vi "get_total_number_of_lines_per_frame.vi"(8 "error in (no error)":errorcluster, 11 "TrajectoryAK101022Resonance in":refnum<class "TrajectoryAK101022Resonance.lvclass">) -> (0 "error out":errorcluster, 2 "total number of lines per frame":i32, 3 "TrajectoryAK101022Resonance out":refnum<class "TrajectoryAK101022Resonance.lvclass">)   [LabVIEW 2010, in "TrajectoryAK101022Resonance.lvclass"]
uses:
  TrajectoryAK101022Resonance.lvclass
  TrajectoryAK101022Resonance.lvclass/TrajectoryAK101022Resonance.ctl
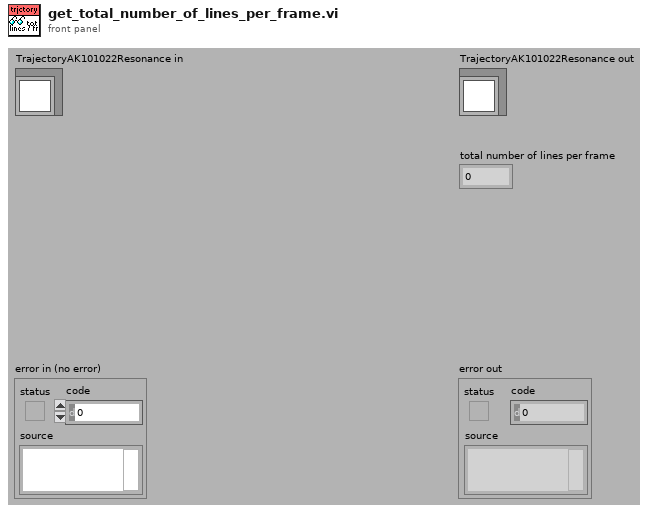
[diagram p1: front panel]
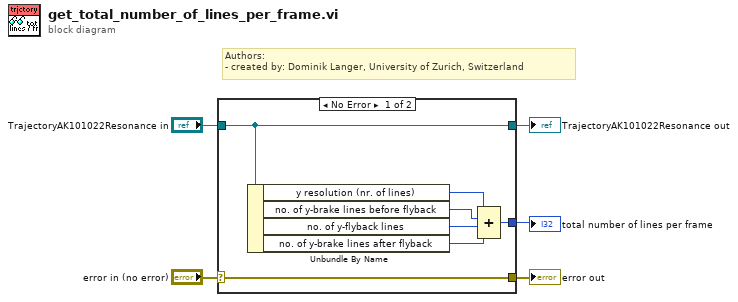
[diagram p0: block diagram]
diagram:
  # "Authors: \n- created by: Dominik Langer, University of Zurich, Switzerland"
  n1 = case shown="No Error" "error in (no error)" {
    selector: "error in (no error)" -> [w12 w14]
    tunnel: [w12 w14] -> w4
    tunnel: [w11 w13] -> w2
    tunnel: "TrajectoryAK101022Resonance in" -> [w11 w13]
    tunnel: [w6 _] -> w1
    frame No Error {
      n2 = Unbundle By Name(w11) -> ("y resolution (nr. of lines)"=w10:i32, "no. of y-brake lines before flyback"=w9:i32, "no. of y-flyback lines"=w8:i32, "no. of y-brake lines after flyback"=w7:i32)
      n3 = Compound Arithmetic op=ADD(w10, w9, w8, w7) -> (w6:i32)
    }
    frame Error {
    }
  }
  "error out" <- w4
  "TrajectoryAK101022Resonance out" <- w2
  "total number of lines per frame" <- w1
